vi "Read En Face.vi"(8 "error in (no error)":errorcluster, 11 "Intensity Processing in":refnum<class "Intensity Processing.lvclass">) -> (0 "error out":errorcluster, 2 "En Face":sgl[][](array[numeric]), 3 "Intensity Processing out":refnum<class "Intensity Processing.lvclass">)   [LabVIEW 2015, in "Intensity Processing.lvclass"]
uses:
  Intensity Processing.lvclass
  Intensity Processing.lvclass/Intensity Processing.ctl
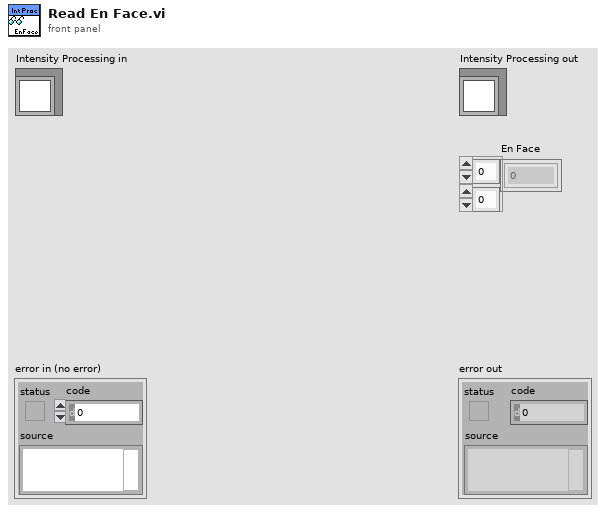
[diagram p1: front panel]
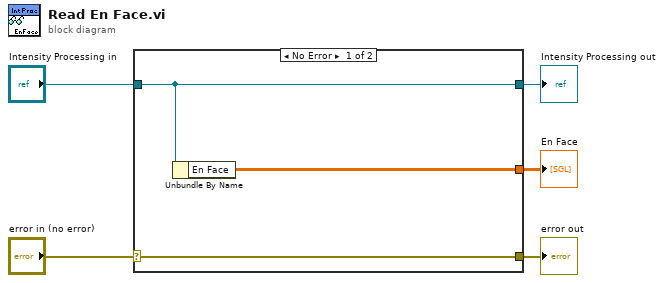
[diagram p0: block diagram]
diagram:
  n1 = case shown="No Error" "error in (no error)" {
    selector: "error in (no error)" -> [w8 w9]
    tunnel: [w8 w9] -> w4
    tunnel: [w7 w10] -> w2
    tunnel: "Intensity Processing in" -> [w7 w10]
    tunnel: [w6 _] -> w1
    frame No Error {
      n2 = Unbundle By Name(w7) -> ("En Face"=w6:sgl[][])
    }
    frame Error {
    }
  }
  "error out" <- w4
  "Intensity Processing out" <- w2
  "En Face" <- w1
